vi "vibrate_GWN.vi"() -> ()   [LabVIEW 2014]
panel:
  in  "Correlation Time (s)":dbl
  in  "Sigma (uW/mm^2)":dbl
  in  "Offset duty cycle":dbl
  in  "Max duty cycle":dbl
  in  "Min duty cycle":dbl
  in  "Frequency (Hz)":dbl
  in  "Frames":i32
  in  "Transfer and Run Date Folder After Experiment":bool
  in  "SSH user name":string
  in  "SSH password":string
  in  "Wait before recording (s)":dbl
  in  "Tags":string
  in  "Start Recording":bool
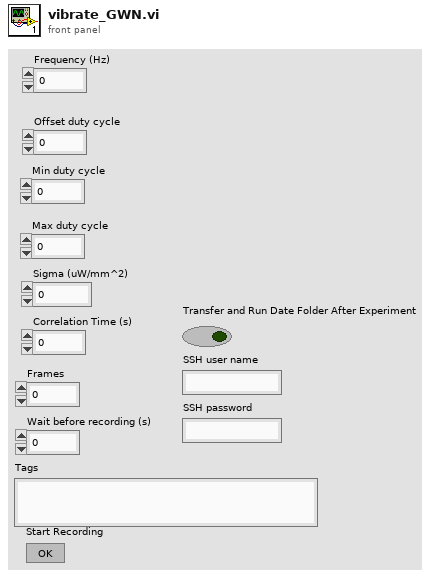
[diagram p1: front panel]
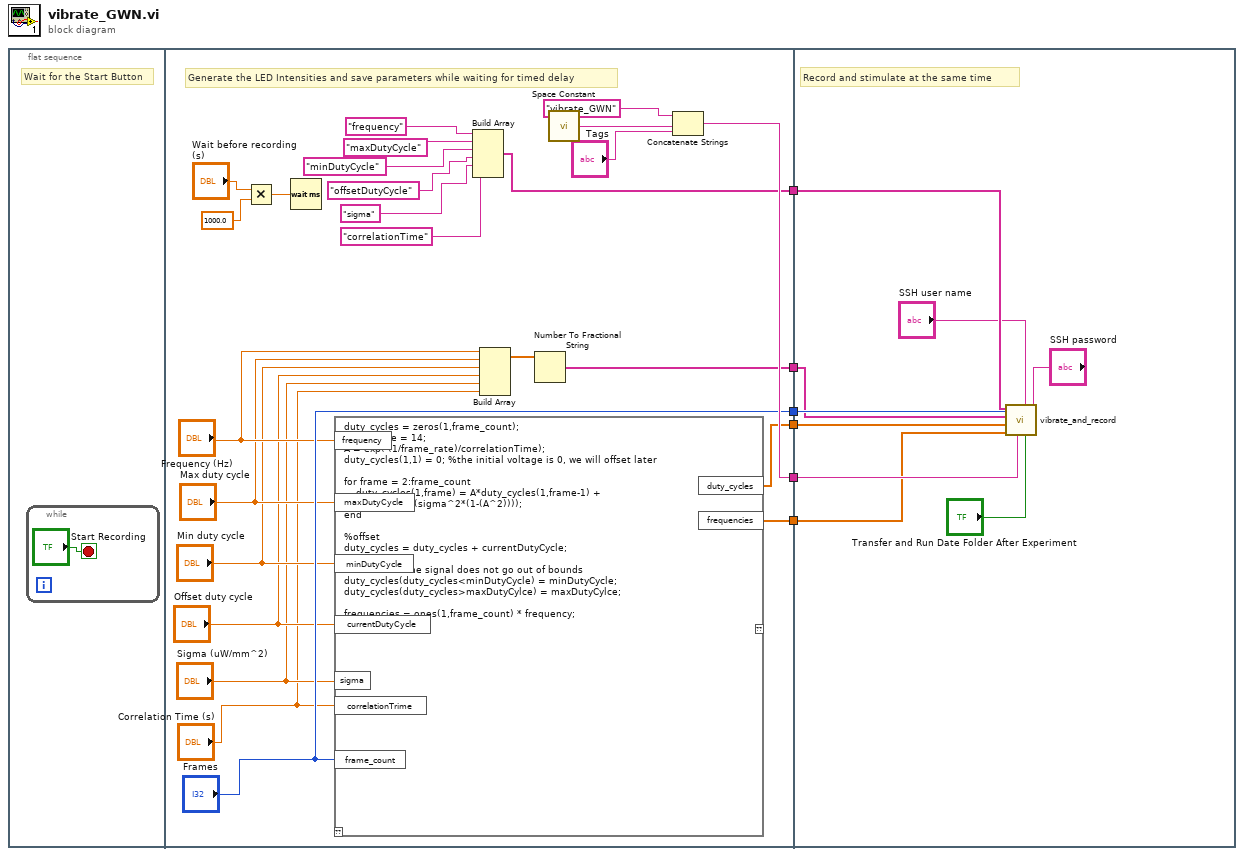
[diagram p0: block diagram]
diagram:
  n1 = flat-sequence {
    tunnel: [w29] -> w6
    tunnel: [w22] -> w5
    tunnel: ["Frames"] -> w4
    tunnel: [w18] -> w3
    tunnel: [w12] -> w2
    tunnel: [w11] -> w1
    tunnel: w6 -> [w41]
    tunnel: w5 -> [w40]
    tunnel: w4 -> [w36]
    tunnel: w3 -> [w35]
    tunnel: w2 -> [w34]
    tunnel: w1 -> [w33]
    frame #0 {
      # "Wait for the Start Button"
      n2 = while {
        stop <- "Start Recording" stop-if-true
      }
    }
    frame #1 {
      # "Generate the LED Intensities and save parameters while waiting for timed delay"
      n3 = Multiply(x="Wait before recording (s)", y=1000.0) -> (x*y=w27:dbl)
      n4 = Wait (ms)(milliseconds to wait=w27) -> ()  [unwired: 1 out]
      n5 = script code="duty_cycles = zeros(1,frame_count);\nframe_rate = 14;\nA = exp(-(1/frame_rate)/correlationTime);\nduty_cycles(1,1) = 0; %the initial voltage is 0, we will offset later\n\nfor frame = 2:frame_count\n    duty_cycles(1,frame) = A*duty_cycles(1,frame-1) + (randn(1)*sqrt(sigma^2*(1-(A^2))));\nend\n\n%offset\nduty_cycles = duty_cycles + currentDutyCycle;\n\n%make sure the signal does not go out of bounds\nduty_cycles(duty_cycles<minDutyCycle) = minDutyCycle;\nduty_cycles(duty_cycles>maxDutyCylce) = maxDutyCylce;\n\nfrequencies = ones(1,frame_count) * frequency;"("currentDutyCycle"="Offset duty cycle", "frame_count"="Frames", "minDutyCycle"="Min duty cycle", "maxDutyCycle"="Max duty cycle", "sigma"="Sigma (uW/mm^2)", "frequency"="Frequency (Hz)", "correlationTrime"="Correlation Time (s)") -> ("duty_cycles"=w12:dbl[], "frequencies"=w11:dbl[])  [unwired: 1 in, 1 out]
      n6 = Build Array("frequency", "maxDutyCycle", "minDutyCycle", "offsetDutyCycle", "sigma", "correlationTime") -> (w22:string[])
      n7 = Build Array("Frequency (Hz)", "Max duty cycle", "Min duty cycle", "Offset duty cycle", "Sigma (uW/mm^2)", "Correlation Time (s)") -> (w17:dbl[])
      n8 = Number To Fractional String(number=w17) -> (F-format string=w18:string[])  [unwired: 3 in]
      n9 = call <vilib>:"Space Constant.vi"() -> ("String"=w31:string)
      n10 = Concatenate Strings("vibrate_GWN", w31, "Tags") -> (w29:string)
    }
    frame #2 {
      # "Record and stimulate at the same time"
      n11 = call "vibrate_and_record.vi"("SSH password"="SSH password", "Transfer and Run Date Folder After Experiment"="Transfer and Run Date Folder After Experiment", "SSH user name"="SSH user name", "Tags"=w41, "Frames"=w36, "frequencies"=w33, "PWM duty cycles"=w34, "parameters"=w35, "parameters headers"=w40) -> ()  [unwired: 3 in]
    }
  }
